vi "Update XY Graph.vi"(8 "error in (no error)":errorcluster, 11 "Top Level in":refnum<class "Top Level.lvclass">) -> (0 "error out":errorcluster, 3 "Top Level out":refnum<class "Top Level.lvclass">)   [LabVIEW 2021, in "Top Level.lvlib" / "Top Level.lvclass"]
uses:
  Top Level.lvclass
  Top Level.lvclass/Top Level.ctl
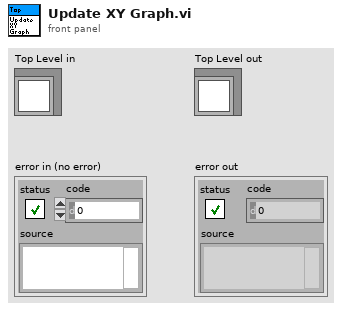
[diagram p1: front panel]
types:
  T1 = cluster{"Voltage To Diode":dbl[], "Voltage Across Diode":dbl[]}
  T2 = cluster{"Voltage To Diode":dbl[], "Current Through Diode":dbl[]}
  T3 = cluster{"Voltage To Diode":dbl[], "Temperature Of Diode":dbl[]}
  T4 = cluster{"Voltage To Diode":dbl[], "Temperature Of Diode":dbl[]}[]
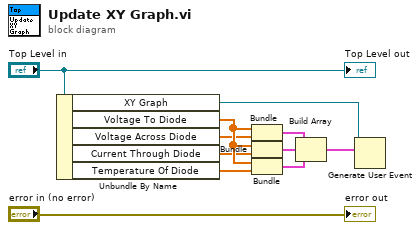
[diagram p0: block diagram]
diagram:
  n1 = Unbundle By Name("Top Level in") -> ("XY Graph"=w10:refnum<user-event>, "Voltage To Diode"=w5:dbl[], "Voltage Across Diode"=w4:dbl[], "Current Through Diode"=w3:dbl[], "Temperature Of Diode"=w2:dbl[])
  n2 = Bundle("Voltage To Diode"=w5, "Voltage Across Diode"=w4) -> (w9:T1)  [unwired: 1 in]
  n3 = Bundle("Voltage To Diode"=w5, "Current Through Diode"=w3) -> (w8:T2)  [unwired: 1 in]
  n4 = Bundle("Voltage To Diode"=w5, "Temperature Of Diode"=w2) -> (w7:T3)  [unwired: 1 in]
  n5 = Build Array(w9, w8, w7) -> (w6:T4)
  n6 = Generate User Event(user event=w10, event data cluster=w6) -> ()  [unwired: 2 in, 2 out]
  "error out" <- "error in (no error)"
  "Top Level out" <- "Top Level in"
